vi "CLSSignalIDMakerConstant.vi"() -> (2 "SignalID":i32[](array[numeric]))   [LabVIEW 2015]
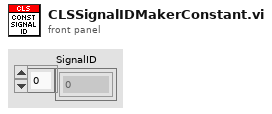
[diagram p1: front panel]
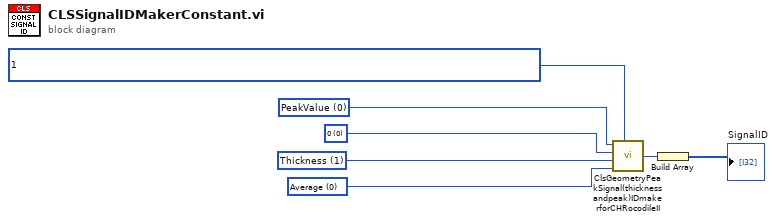
[diagram p0: block diagram]
diagram:
  w7 = 0 items=["Average"=0, "Standard Deviation"=1, "Minimum"=3, "Maximum"=4, "Peak-to-peak (max-min)"=5] ("Statistics for a given\naveraging period\n(set by AVD):")
  w6 = 1 items=["Peak", "Thickness"] ("Combination(peak or thickness)")
  w5 = 0 items=["0", "1", "2", "3", "4", "5", "6", "7", "8", "9", "10", "11", "12", "13", "14", "15"] ("Peak Index(no more than 4 for multiple channel devices)")
  w4 = 0 items=["PeakValue"=0, "PeakValue Median"=4, "PeakWidth"=5] ("Peak Signal Name")
  n1 = call "ClsGeometryPeakSignal(thicknessandpeak)IDmakerforCHRocodileII.vi"("Peak Signal Name"=w4, "Peak Index(no more than 4 for multiple channel devices)"=w5, "Combination(peak or thickness)"=w6, "Statistics for a given\naveraging period\n(set by AVD):"=w7, "Value Encoding(Geometric: distance and thickness)"=1) -> ("Peak Signal ID"=w2:i32)
  n2 = Build Array(w2) -> (→"SignalID":i32[])
